vi "Sequence numbering.vi"(11 "Item Names IN":string[](array[string])=["Wait for 11 s", "Run Macro C:\\Users\\shared\\NML Data Acquisition\\monovu\\sub1.txt", "Wait for 131 s", "Run Macro C:\\Users\\shared\\NML Data Acquisition\\monovu\\sub2.txt", "Wait for 131 s", "END SEQUENCE"]) -> (2 "unnested items":string[](array[string])=["Wait for 11 s", "Wait for 2.1 s", "Wait for 2.2 s", "Wait for 2.3 s", "Wait for 3 s", "----------    end of sequence line removed", "----------    end of sequence line removed", "----------    end of sequence line removed", "----------    end of sequence line removed", "END SUBsequence", "Wait for 131 s", "Wait for 2.2 s", "Wait for 2.3 s", "Wait for 3 s", "----------    end of sequence line removed", "----------    end of sequence line removed", "----------    end of sequence line removed", "END SUBsequence", "Wait for 131 s", "END SEQUENCE"], 3 "item index":string[](array[string])=["0.0", "1.0", "1.1", "1.2", "1.3", "1.4", "1.5", "1.6", "1.7", "1.8", "2.0", "3.0", "3.1", "3.2", "3.3", "3.4", "3.5", "3.6", "4.0", "5.0"])   [LabVIEW 2025]
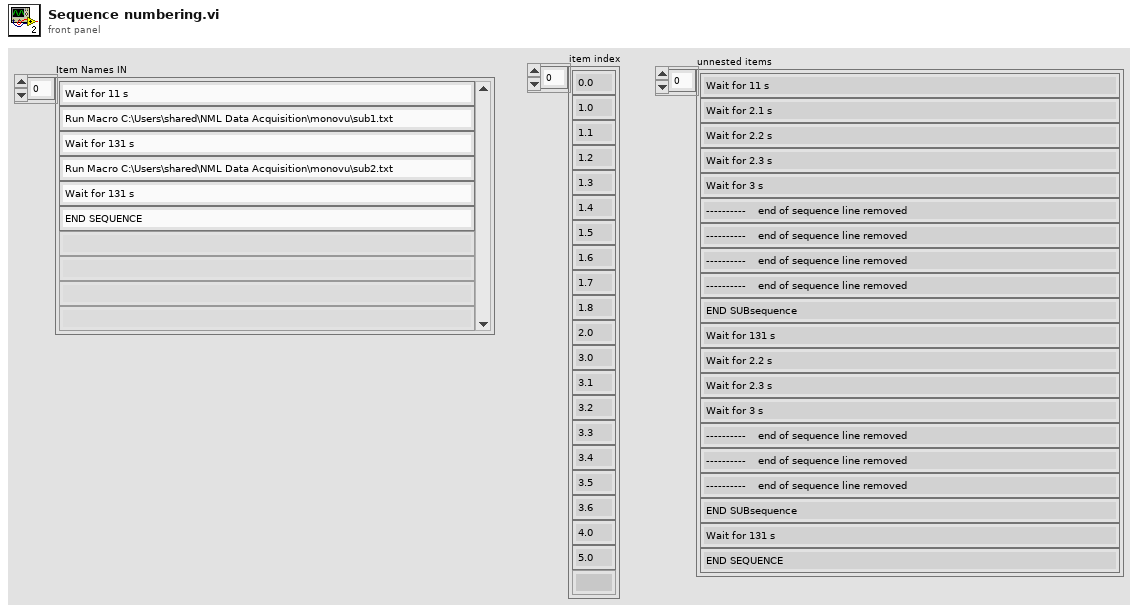
[diagram p1: front panel]
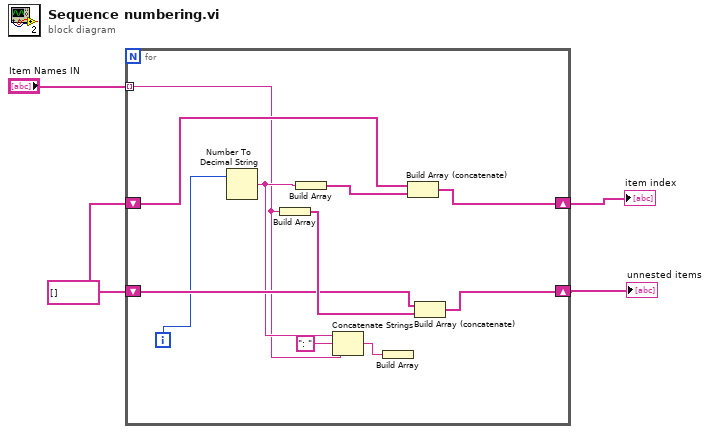
[diagram p0: block diagram]
diagram:
  w3 = string[] []
  n1 = for {
    tunnel: "Item Names IN" -> [w6] mode=indexing
    shift-right: [w14] -> w1
    shift-left: w3 -> [w13]
    shift-right: [w10] -> w2
    shift-left: w3 -> [w9]
    i -> [w12]
    n2 = Number To Decimal String(number=w12) -> (decimal integer string=w8:string)  [unwired: 1 in]
    n3 = Build Array(w6) -> (w15:string[])
    n4 = Build Array(w8) -> (w11:string[])
    n5 = Concatenate Strings(w8, ": " ("string"), w6) -> (w5:string)
    n6 = Build Array(w5) -> ()  [unwired: 1 out]
    n7 = Build Array (concatenate)(w9, w11) -> (w10:string[])
    n8 = Build Array (concatenate)(w13, w15) -> (w14:string[])
  }
  "item index" <- w2
  "unnested items" <- w1
